vi "ex2.vi"() -> ()   [LabVIEW 2021]
uses:
  <vilib>/Analysis/5stat.llb/RMS (DBL).vi
  <vilib>/Analysis/NI_AALPro.lvlib
panel:
  out "rms value Channel 1":dbl format="%0.2f"
  out "rms value Channel 0":dbl format="%0.2f"
  out "Waveform Graph":dbl[][](graph)
  in  "Amplitude":dbl
  in  "Number of Samples":dbl
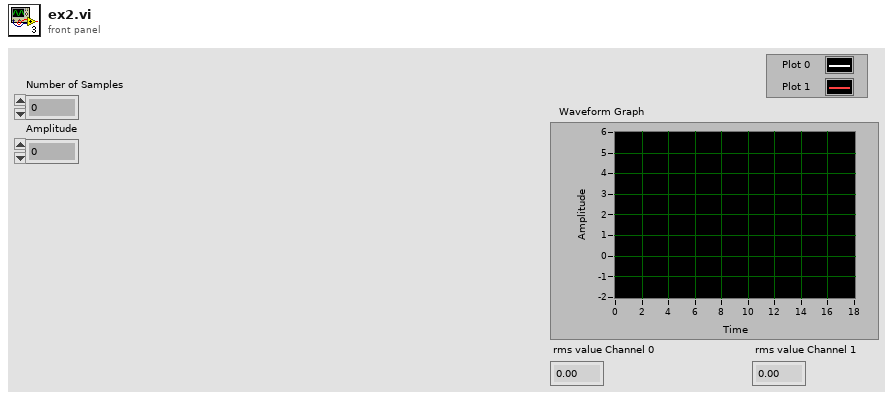
[diagram p1: front panel]
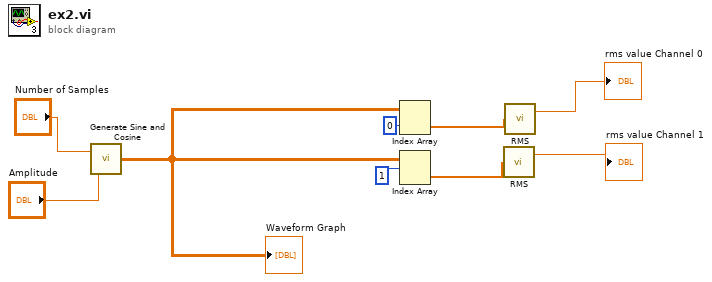
[diagram p0: block diagram]
diagram:
  n1 = call "Generate Sine and Cosine.vi"("Amplitude"="Amplitude", "Number of Samples"="Number of Samples") -> ("Waveform Graph"=w3:dbl[][])
  "Waveform Graph" <- w3
  n2 = Index Array(array=w3, index (row)=0 ("index")) -> (element=w2:dbl[])  [unwired: 1 in]
  n3 = Index Array(array=w3, index (row)=1 ("index")) -> (element=w1:dbl[])  [unwired: 1 in]
  n4 = call-poly <vilib>:"RMS.vi"("X"=w1) -> ("rms value"=→"rms value Channel 1":dbl)  [unwired: 1 out]
  n5 = call-poly <vilib>:"RMS.vi"("X"=w2) -> ("rms value"=→"rms value Channel 0":dbl)  [unwired: 1 out]
